vi "stopped.vi"(8 "error in (no error)":errorcluster, 10 "HWloop":bool, 11 "ExperimentControl in":refnum<class "ExperimentControl.lvclass">) -> (0 "error out":errorcluster, 1 "stoppedByUser":bool, 2 "stopBeforeNext":bool, 3 "ExperimentControl out":refnum<class "ExperimentControl.lvclass">)   [LabVIEW 2011, in "Views.lvlib" / "ExperimentControl.lvlib" / "ExperimentControl.lvclass"]
uses:
  ExperimentControl.lvclass
  ExperimentControl.lvclass/ExperimentControl.ctl
  Events/Event.lvclass
  Events/ExperimentControlEvents.lvclass
  Hal/HWController/HWControllerEvents/HWControllerEvents.lvclass
panel:
  out "element":T1(ring)
  out "stopUser":bool
  out "stopHW":bool
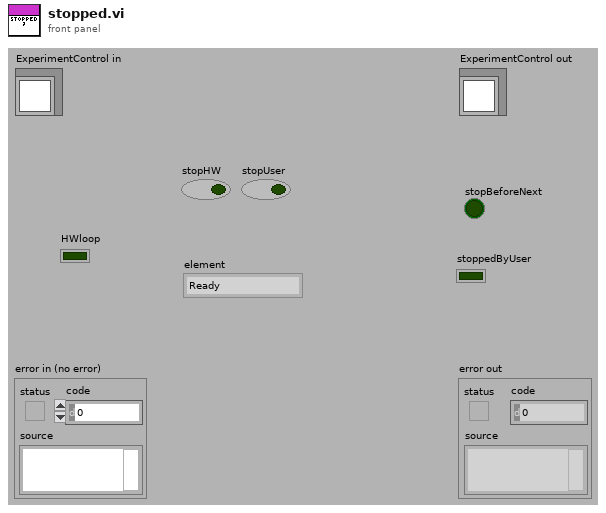
[diagram p1: front panel]
types:
  T1 = enum16{"Ready", "Compiling", "Configured", "Running", "Stopping", "Unresolved Error"}
  T2 = cluster{"incomingEventTypes":cluster{"start":cluster{"Boolean":bool}, "stop":cluster{"Boolean":bool}, "statusInquiry":cluster{"Boolean":bool}, "configure":cluster{"DPScriptPath":path, "TimeStamp":string, "HWLoop?":bool}, "resetError":cluster{"Boolean":bool}, "resourcesInquiry":cluster{"Boolean":bool}, "reserveResources":cluster{"HWList":string[]}, "initialise":cluster{"HWList":string[]}, "close":cluster{"Boolean":bool}, "resetAllChannels":cluster{"Boolean":bool}, "staticChannelUpdate":cluster{"channel_address":string, "calibratedValue":dbl}, "runScript":cluster{"DPScriptPath":path, "TimeStamp":string, "HWLoop?":bool}, "compilingScript":cluster{"Path":path}, "compiledScript":cluster{"Path":path, "timeCompileAt":string}, "compilerError":cluster{"Path":path}, "configureCompiledScript":cluster{"DPScriptPath":path, "TimeStamp":string, "HWLoop?":bool, "CompiledScript":cluster{"ScriptListCompiler.lvclass":refnum<class "ScriptListCompiler.lvclass">, "aoChannels":refnum<class "AnalogOutput.lvclass">[], "doChannels":refnum<class "DigitalOutput.lvclass">[], "rfChannels":refnum<class "DDSOutput.lvclass">[]}}, "restartCompiler":cluster{"restart":bool}, "staticRfChannelUpdate":cluster{"channel_address":string, "Output":cluster{"Frequency(MHz)":dbl, "Amplitude":dbl, "Phase":dbl, "OutputForm":enum16{"Sine", "Square", "Triangle", "Arbitrary"}}}, "cameraUpdate":cluster{"Camera":string, "Type":string, "settings":path}}, "outgoingEventTypes":cluster{"HWStatus":cluster{"status":enum16{"Ready", "Compiling", "Configured", "Running", "Stopping", "Unresolved Error"}}, "error":cluster{"error out":errorcluster}, "resourcesAvailable":cluster{"availableHWList":string[], "reservedHWList":string[]}, "resourcesReserved":cluster{"reservedHWList":string[]}}}
  T3 = cluster{"status":enum16{"Ready", "Compiling", "Configured", "Running", "Stopping", "Unresolved Error"}}
  T4 = enum16{"start", "stop", "statusInquiry", "configure", "resetError", "resourcesInquiry", "reserveResources", "initialise", "resetAllChannels", "staticUpdate", "close", "HWStatus", "error", "resourcesAvailable", "resourcesReserved", "compilerError", "compiledScript", "compilingScript", "runScript", "configureCompiledScript", "restartCompiler", "staticRfChannelUpdate", "cameraUpdate"}
  T5 = enum16{"close", "stopRunning", "runSingleScript", "runExperiment", "runExperimentScript", "Unregistered", "hasStopped"}
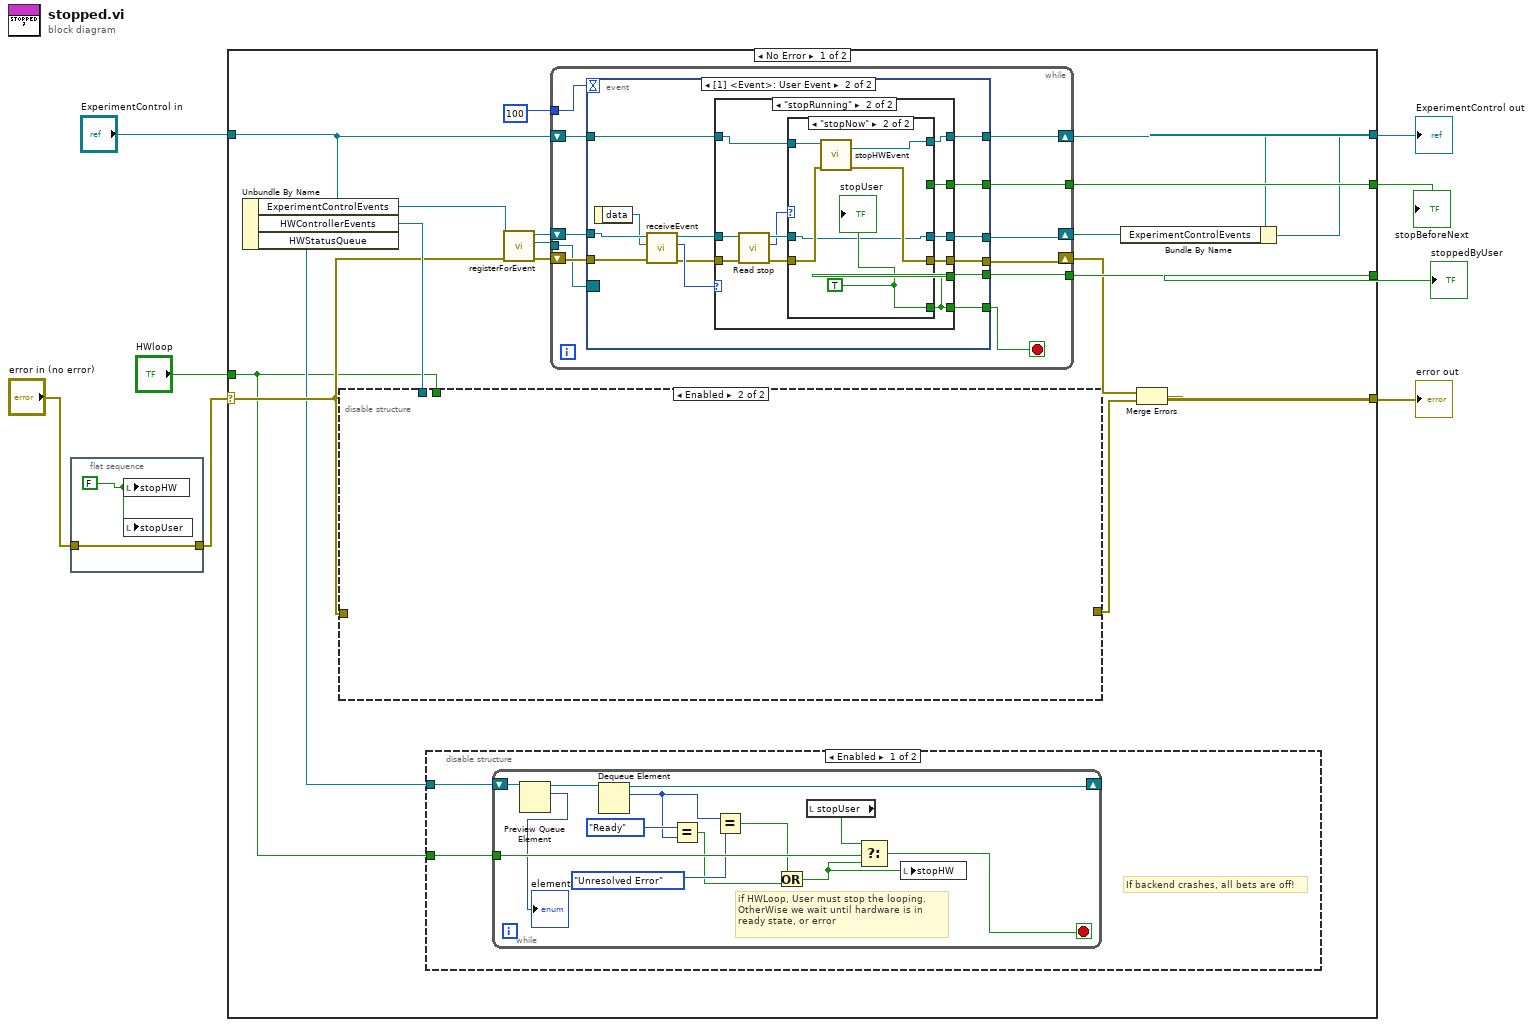
[diagram p0: block diagram]
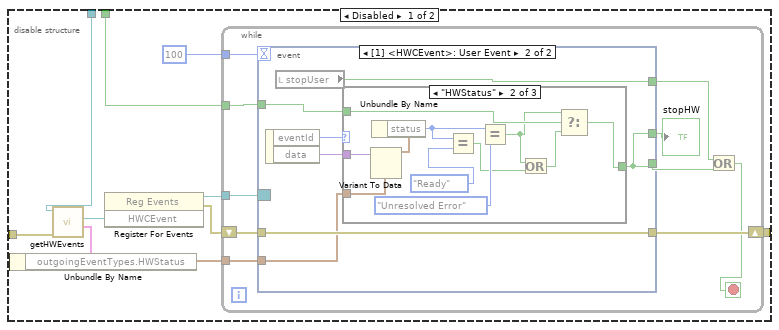
[diagram p3: hidden frame]
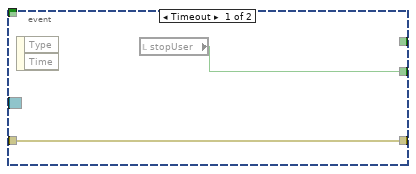
[diagram p4: hidden frame]
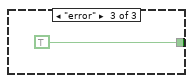
[diagram p6: hidden frame]
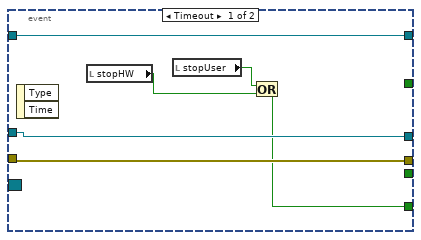
[diagram p7: hidden frame]
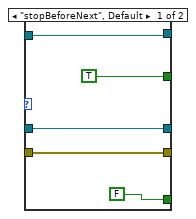
[diagram p9: hidden frame]
diagram:
  n1 = flat-sequence {
    tunnel: "error in (no error)" -> [w9]
    tunnel: [w9] -> w3
    frame #0 {
      w10 = FALSE
      n2 = local write "stopHW"(w10) -> ()
      n3 = local write "stopUser"(w10) -> ()
    }
  }
  n4 = case shown="No Error" w3 {
    selector: w3 -> [w22 w141]
    tunnel: [w17 w141] -> w8
    tunnel: [w13 w140] -> w6
    tunnel: "ExperimentControl in" -> [w28 w140]
    tunnel: [w20 _] -> w5
    tunnel: [w16 _] -> w2
    tunnel: "HWloop" -> [w11 _]
    frame No Error {
      n5 = Unbundle By Name(w28) -> ("ExperimentControlEvents"=w27:refnum<class "ExperimentControlEvents.lvclass">, "HWControllerEvents"=w23:refnum<class "HWControllerEvents.lvclass">, "HWStatusQueue"=w12:refnum<queue>)
      n6 = disable-structure shown="Enabled" {
        disable-tunnel: w23 -> [w52 _]
        disable-tunnel: w22 -> [w51 _]
        disable-tunnel: [w45 _] -> w18
        disable-tunnel: w11 -> [w44 _]
        frame Disabled {
          n7 = call-dynamic "getHWEvents.vi"("error in (no error)"=w51, "HWControllerEvents in"=w52) -> ("eventDataTypes"=w48:T2, "HWCEvent"=w53:refnum<user-event>)  [unwired: 6 in, 2 out]
          n8 = Unbundle By Name(w48) -> ("outgoingEventTypes.HWStatus"=w47:T3)
          n9 = register-events(w53) -> (reference out=w50:refnum<event-registration>, error out=w49:errorcluster)  [unwired: 2 in]
          n10 = while {
            shift-right: [w62] -> w45
            shift-left: w49 -> [w61]
            tunnel: w50 -> [w63]
            tunnel: w47 -> [w60]
            tunnel: 100 -> [w59]
            tunnel: w44 -> [w55]
            stop <- w54 stop-if-true
            n11 = event shown="[1] <HWCEvent>: User Event" {
              selector: w63 -> [_ _]
              dyn-events: _ -> [_ _]
              timeout: w59 -> [_ _]
              tunnel: [w65 w72] -> w62
              tunnel: w61 -> [w65 w72]
              tunnel: w60 -> [_ w69]
              tunnel: [w64 w68] -> w56
              tunnel: [_ w68] -> w58
              tunnel: [_ w67] -> w57
              tunnel: w55 -> [_ w66]
              event Timeout {
                n12 = event-data() -> ()  [unwired: 1 in, 2 out]
                n13 = local read "stopUser"() -> (w64:bool)
              }
              event User Event {
                n14 = event-data() -> ("eventId"=w71:T4, "data"=w70:variant)  [unwired: 1 in]
                n15 = local read "stopUser"() -> (w67:bool)
                n16 = case shown="\"HWStatus\"" w71 {
                  tunnel: w70 -> [_ w83 _]
                  tunnel: w69 -> [_ w82 _]
                  tunnel: [_ w73 TRUE] -> w68
                  tunnel: w66 -> [_ w76 _]
                  frame Default {
                  }
                  frame "HWStatus" {
                    n17 = Variant To Data(type=w82, Variant=w83) -> (data=w81:T3)  [unwired: 1 in, 1 out]
                    n18 = Unbundle By Name(w81) -> ("status"=w79:T1)
                    n19 = Equal?(x=w79, y=T1."Ready" ("status")) -> (x = y?=w77:bool)
                    n20 = Equal?(x=w79, y=T1."Unresolved Error" ("status")) -> (x = y?=w75:bool)
                    n21 = Or(x=w75, y=w77) -> (x .or. y?=w74:bool)
                    n22 = Select(t=w75, s=w76, f=w74) -> (s? t:f=w73:bool)
                  }
                  frame "error" {
                  }
                }
              }
            }
            "stopHW" <- w58
            n23 = Or(x=w57, y=w56) -> (x .or. y?=w54:bool)
          }
        }
        frame Enabled {
        }
      }
      n24 = disable-structure shown="Enabled" {
        disable-tunnel: w12 -> [w30 _]
        disable-tunnel: w11 -> [w29 _]
        frame Enabled {
          # "If backend crashes, all bets are off!"
          n25 = while {
            tunnel: w29 -> [w41]
            shift-right: [w42] -> _
            shift-left: w30 -> [w43]
            stop <- w34 stop-if-true
            # "if HWLoop, User must stop the looping.\nOtherWise we wait until hardware is in \nready state, or error"
            n26 = Preview Queue Element(queue=w43) -> (queue out=w32:refnum<queue>, element=→"element":T1)  [unwired: 2 in, 2 out]
            n27 = Dequeue Element(queue=w32) -> (queue out=w42:refnum<queue>, element=w39:T1)  [unwired: 2 in, 2 out]
            n28 = Equal?(x=T1."Ready" ("status"), y=w39) -> (x = y?=w36:bool)
            n29 = Equal?(x=w39, y=T1."Unresolved Error" ("status")) -> (x = y?=w37:bool)
            n30 = Or(x=w37, y=w36) -> (x .or. y?=w33:bool)
            n31 = local read "stopUser"() -> (w35:bool)
            n32 = Select(t=w35, s=w41, f=w33) -> (s? t:f=w34:bool)
            n33 = local write "stopHW"(w33) -> ()
          }
        }
        frame Disabled {
        }
      }
      n34 = call "registerForEvent.vi"("error in (no error)"=w22, "Event in"=w27) -> ("error out"=w25:errorcluster, "Event Registration Refnum"=w24:refnum<event-registration>, "Event out"=w26:refnum<class "ExperimentControlEvents.lvclass">)  [unwired: 6 in, 1 out]
      n35 = while {
        shift-right: [w94] -> w14
        shift-left: w28 -> [w95]
        shift-right: [w89] -> w15
        shift-left: w26 -> [w93]
        shift-right: [w90] -> w19
        shift-left: w25 -> [w92]
        tunnel: w24 -> [w91]
        tunnel: 100 -> [w88]
        tunnel: [w86] -> w20
        tunnel: [w85] -> w16
        stop <- w87 stop-if-true
        n36 = event shown="[1] <Event>: User Event" {
          selector: w91 -> [_ _]
          dyn-events: _ -> [_ _]
          timeout: w88 -> [_ _]
          tunnel: w95 -> [w101 w104]
          tunnel: [w101 w103] -> w94
          tunnel: w93 -> [w100 w114]
          tunnel: w92 -> [w99 w112]
          tunnel: [w99 w107] -> w90
          tunnel: [w100 w109] -> w89
          tunnel: [w96 w106] -> w87
          tunnel: [_ w105] -> w86
          tunnel: [_ w102] -> w85
          event Timeout {
            n37 = event-data() -> ()  [unwired: 1 in, 2 out]
            n38 = local read "stopHW"() -> (w97:bool)
            n39 = local read "stopUser"() -> (w98:bool)
            n40 = Or(x=w98, y=w97) -> (x .or. y?=w96:bool)
          }
          event User Event {
            n41 = event-data() -> ("data"=w113:refnum<class>)  [unwired: 1 in]
            n42 = call "receiveEvent.vi"("error in (no error)"=w112, "data"=w113, "ExperimentControlEvents in"=w114) -> ("error out"=w108:errorcluster, "Enum"=w111:T5, "ExperimentControlEvents out"=w110:refnum<class "ExperimentControlEvents.lvclass">)  [unwired: 6 in]
            n43 = case shown="\"stopRunning\"" w111 {
              tunnel: w110 -> [w117 w127]
              tunnel: [w117 w119] -> w109
              tunnel: w108 -> [w116 w126]
              tunnel: [w116 w120] -> w107
              tunnel: [_ w128] -> w106
              tunnel: [_ w128] -> w105
              tunnel: w104 -> [w115 w122]
              tunnel: [w115 w121] -> w103
              tunnel: [_ w118] -> w102
              frame Default {
              }
              frame "stopRunning" {
                n44 = call "Read stop.vi"("error in (no error)"=w126, "ExperimentControlEvents in"=w127) -> ("error out"=w124:errorcluster, "stop"=w123:enum16{"stopBeforeNext", "stopNow"}, "ExperimentControlEvents out"=w125:refnum<class "ExperimentControlEvents.lvclass">)  [unwired: 7 in]
                n45 = case shown="\"stopNow\"" w123 {
                  tunnel: [FALSE w139] -> w128
                  tunnel: w125 -> [w131 w134]
                  tunnel: w124 -> [w133 w136]
                  tunnel: w122 -> [w130 w138]
                  tunnel: [w130 w137] -> w121
                  tunnel: [w133 w135] -> w120
                  tunnel: [w131 w134] -> w119
                  tunnel: [TRUE _] -> w118
                  frame "stopBeforeNext", Default {
                  }
                  frame "stopNow" {
                    w139 = TRUE
                    n46 = call "stopHWEvent.vi"("error in (no error)"=w136, "ExperimentControl in"=w138) -> ("error out"=w135:errorcluster, "ExperimentControl out"=w137:refnum<class "ExperimentControl.lvclass">)  [unwired: 8 in]
                    "stopUser" <- w139
                  }
                }
              }
            }
          }
        }
      }
      n47 = Bundle By Name(cluster=w14, "ExperimentControlEvents"=w15) -> (w13:refnum<class "ExperimentControl.lvclass">)
      n48 = Merge Errors(w19, w18) -> (w17:errorcluster)
    }
    frame Error {
    }
  }
  "error out" <- w8
  "ExperimentControl out" <- w6
  "stoppedByUser" <- w5
  "stopBeforeNext" <- w2
